vi "Example - cmd.vi"() -> ()   [LabVIEW 2019]
uses:
  .NET Process/SystemProcessManager.lvclass
panel:
  in  "Working Directory":path=path "c:/"
  out "ErrOut":string
  out "StdOut":string
  in  "Send":bool
  in  "Cmd In":string="dir"
  in  "Stop":bool
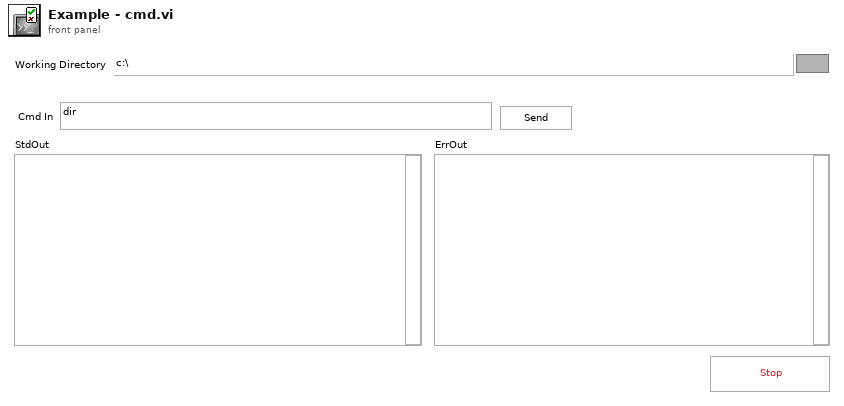
[diagram p1: front panel]
types:
  T1 = cluster{"StdOut Event":refnum<user-event>, "StdErr Event":refnum<user-event>}
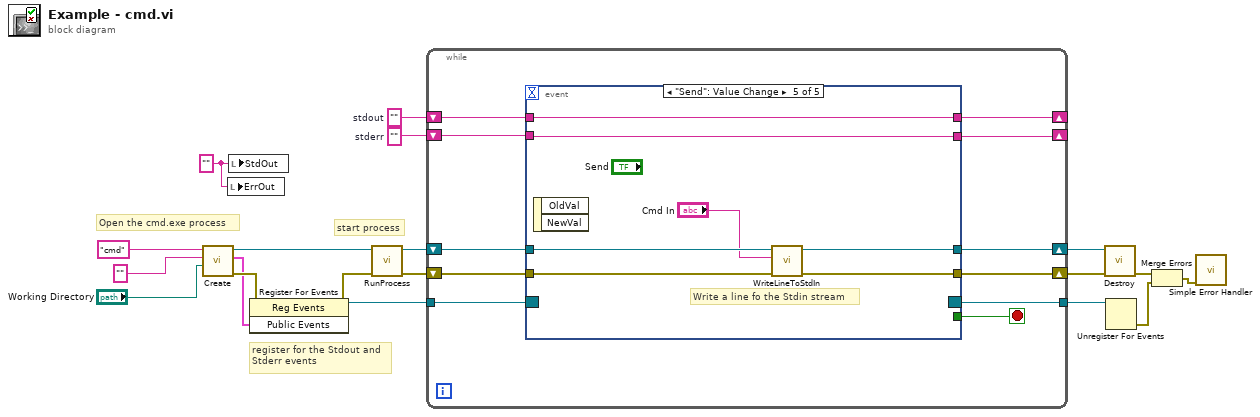
[diagram p0: block diagram]
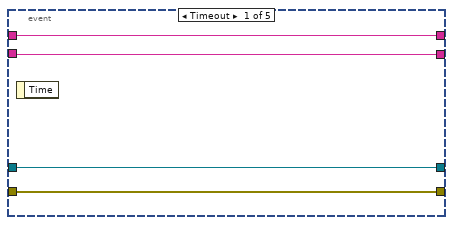
[diagram p2: hidden frame]
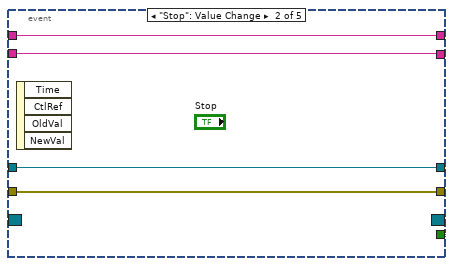
[diagram p3: hidden frame]
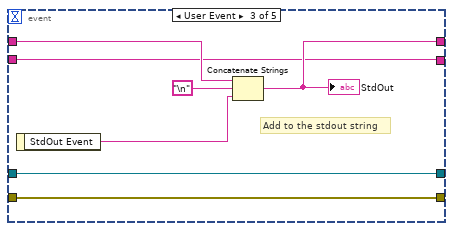
[diagram p4: hidden frame]
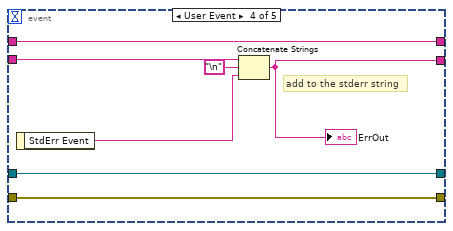
[diagram p5: hidden frame]
diagram:
  w1 = "" ("Process File Name")
  w3 = ""  # stderr
  w9 = ""  # stdout
  # "register for the Stdout and\nStderr events"
  # "start process"
  # "Open the cmd.exe process"
  n1 = call "Create.vi"("Working Directory (blank: current VI's path)"="Working Directory", "Arguments (empty)"="" ("Process File Name"), "Process File Name"="cmd") -> ("error out"=w6:errorcluster, "Public Events"=w4:T1, ".NET Process out"=w17:refnum<class "SystemProcessManager.lvclass">)  [unwired: 6 in]
  n2 = local write "ErrOut"(w1) -> ()
  n3 = local write "StdOut"(w1) -> ()
  n4 = register-events(error in=w6, w4) -> (reference out=w16:refnum<event-registration>, error out=w5:errorcluster)  [unwired: 1 in]
  n5 = call "RunProcess.vi"("error in (no error)"=w5, ".NET Process in"=w17) -> ("error out"=w7:errorcluster, ".NET Process out"=w19:refnum<class "SystemProcessManager.lvclass">)  [unwired: 8 in]
  n6 = while {
    shift-right: [w30] -> w18
    shift-left: w19 -> [w29]
    shift-right: [w27] -> w14
    shift-left: w7 -> [w28]
    tunnel: w16 -> [w26]
    tunnel: [w25] -> w15
    shift-right: [w23] -> _
    shift-left: w9 -> [w24]
    shift-right: [w20] -> _
    shift-left: w3 -> [w21]
    stop <- w22 stop-if-true
    n7 = event shown="[4] \"Send\": Value Change" {
      selector: w26 -> [_ _ _ _ _]
      dyn-events: [_ _ _ _ _] -> w25
      timeout: _ -> [_ _ _ _ _]
      tunnel: [w34 w39 w46 w53 w60] -> w30
      tunnel: w29 -> [w34 w39 w46 w53 w59]
      tunnel: w28 -> [w33 w38 w45 w52 w57]
      tunnel: [w33 w38 w45 w52 w58] -> w27
      tunnel: w24 -> [w32 w36 w42 w48 w55]
      tunnel: [w32 w36 w43 w48 w55] -> w23
      tunnel: [_ TRUE _ _ _] -> w22
      tunnel: w21 -> [w31 w35 w40 w49 w54]
      tunnel: [w31 w35 w40 w47 w54] -> w20
      event Timeout {
        n8 = event-data() -> ()  [unwired: 1 in, 1 out]
      }
      event "Stop": Value Change {
        n9 = event-data() -> ()  [unwired: 1 in, 4 out]
      }
      event User Event {
        # "Add to the stdout string"
        n10 = event-data() -> ("StdOut Event"=w41:string)  [unwired: 1 in]
        n11 = Concatenate Strings(w42, "\n", w41) -> (w43:string)
        "StdOut" <- w43
      }
      event User Event {
        # "add to the stderr string"
        n12 = event-data() -> ("StdErr Event"=w50:string)  [unwired: 1 in]
        n13 = Concatenate Strings(w49, "\n", w50) -> (w47:string)
        "ErrOut" <- w47
      }
      event "Send": Value Change {
        # "Write a line fo the Stdin stream"
        n14 = event-data() -> ()  [unwired: 1 in, 2 out]
        n15 = call-dynamic "WriteLineToStdIn.vi"("error in (no error)"=w57, "Input"="Cmd In", ".NET Process in"=w59) -> ("error out"=w58:errorcluster, ".NET Process out"=w60:refnum<class "SystemProcessManager.lvclass">)  [unwired: 7 in]
      }
    }
  }
  n16 = call-dynamic "Destroy.vi"("error in (no error)"=w14, ".NET Process in"=w18) -> ("error out"=w13:errorcluster)  [unwired: 8 in, 1 out]
  n17 = Unregister For Events(event registration refnum=w15) -> (error out=w12:errorcluster)  [unwired: 1 in]
  n18 = Merge Errors(w13, w12) -> (w11:errorcluster)
  n19 = call <vilib>:"Simple Error Handler.vi"("error in (no error)"=w11) -> ()  [unwired: 4 in, 5 out]
